vi "运维调试.vi"() -> ()   [LabVIEW 2016]
uses:
  <vilib>/Utility/miscctls.llb/LVPointTypeDef.ctl
  PLC/PLC.lvlib
panel:
  in  "运维调试单选按钮":enum32{"采配水", "CodCr", "总磷氨氮", "pH", "其他"}(xcontrol)
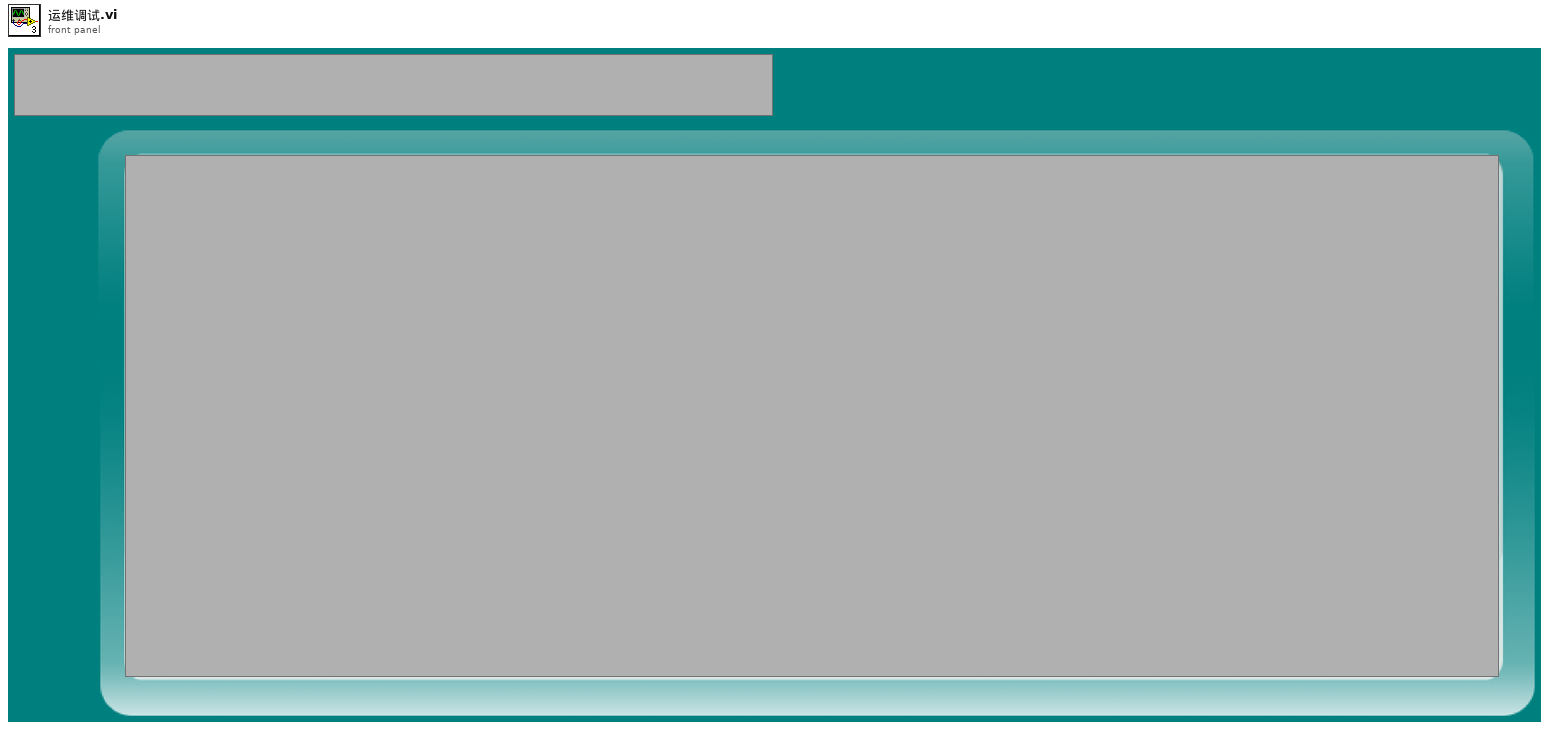
[diagram p1: front panel]
types:
  T1 = typedef "LVPointTypeDef.ctl" = cluster{"Horizontal":i16, "Vertical":i16}
  T2 = enum32{"Bad", "Idle", "Run top level", "Running"}
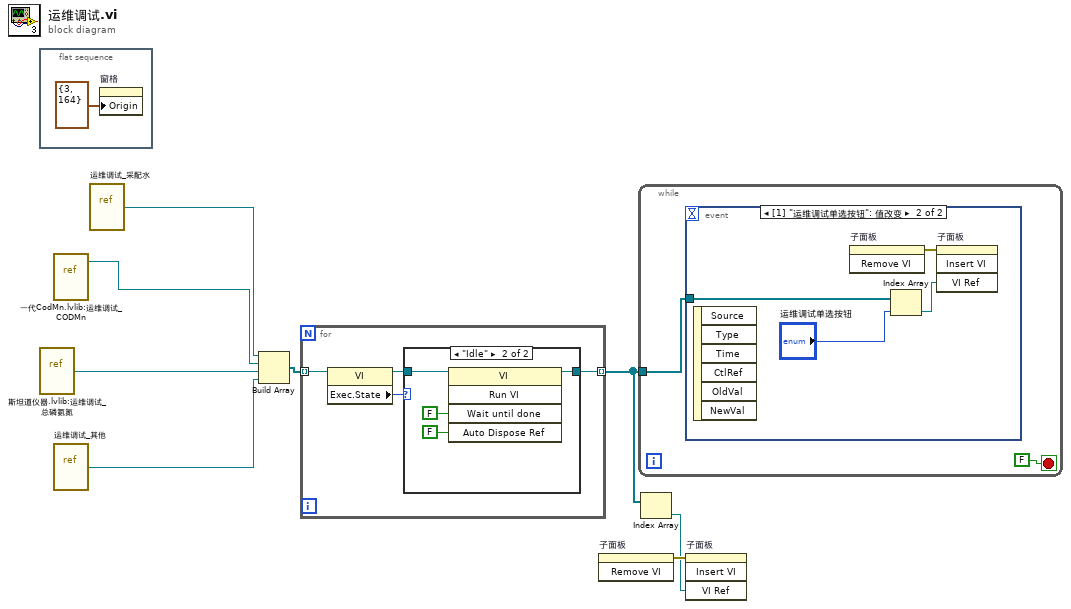
[diagram p0: block diagram]
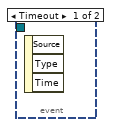
[diagram p3: hidden frame]
diagram:
  n1 = flat-sequence {
    frame #0 {
      n2 = property on="窗格" class="Pane"("Origin"=T1 {"Horizontal"=3, "Vertical"=164} ("原点")) -> ()  [unwired: 2 in, 2 out]
    }
  }
  n3 = vi-ref "斯坦道仪器.lvlib:运维调试_总磷氨氮.vi"() -> (w3:refnum<vi>)
  n4 = vi-ref "一代CodMn.lvlib:运维调试_CODMn.vi"() -> (w1:refnum<vi>)
  n5 = vi-ref "运维调试_其他.vi"() -> (w2:refnum<vi>)
  n6 = vi-ref "运维调试_采配水.vi"() -> (w5:refnum<vi>)
  n7 = Build Array(w5, w1, w3, w2) -> (w4:refnum<vi>[])
  n8 = for {
    tunnel: w4 -> [w13] mode=indexing
    tunnel: [w10] -> w7 mode=indexing
    n9 = property class="VI"(reference=w13) -> (reference out=w11:refnum<vi>, "Exec.State"=w12:T2)  [unwired: 1 in, 1 out]
    n10 = case shown="\"Idle\"" w12 {
      tunnel: w11 -> [w14 w16]
      tunnel: [w14 w15] -> w10
      frame "Bad", Default {
      }
      frame "Idle" {
        n11 = invoke class="VI" method="Run VI"(reference=w16, "Wait until done"=FALSE ("结束前等待"), "Auto Dispose Ref"=FALSE ("自动销毁引用")) -> (reference out=w15:refnum<vi>)  [unwired: 2 in, 4 out]
      }
    }
  }
  n12 = invoke on="子面板" class="SubPnl" method="Remove VI"() -> (error out=w8:errorcluster)  [unwired: 3 in, 2 out]
  n13 = while {
    tunnel: w7 -> [w19]
    stop <- FALSE stop-if-true
    n14 = event shown="[1] \"运维调试单选按钮\": 值改变" {
      selector: _ -> [_ _]
      dyn-events: _ -> [_ _]
      timeout: _ -> [_ _]
      tunnel: w19 -> [_ w22]
      event Timeout {
        n15 = event-data() -> ()  [unwired: 1 in, 3 out]
      }
      event "运维调试单选按钮": Value Change {
        n16 = event-data() -> ()  [unwired: 1 in, 6 out]
        n17 = invoke on="子面板" class="SubPnl" method="Remove VI"() -> (error out=w24:errorcluster)  [unwired: 3 in, 2 out]
        n18 = Index Array(array=w22, index="运维调试单选按钮") -> (element=w21:refnum<vi>)
        n19 = invoke on="子面板" class="SubPnl" method="Insert VI"(error in=w24, "VI Ref"=w21) -> ()  [unwired: 2 in, 4 out]
      }
    }
  }
  n20 = Index Array(array=w7) -> (element=w6:refnum<vi>)  [unwired: 1 in]
  n21 = invoke on="子面板" class="SubPnl" method="Insert VI"(error in=w8, "VI Ref"=w6) -> ()  [unwired: 2 in, 4 out]
